vi "QR Code_Example.vi"() -> ()   [LabVIEW 2016]
uses:
  Data Def/QR Code_QR Code Setting.ctl
  <vilib>/vision/Instrument.llb/QR Code Search Options.ctl
  <vilib>/vision/Instrument.llb/Demodulation Mode.ctl
  <vilib>/vision/Instrument.llb/Cell Sample Size.ctl
  <vilib>/vision/Instrument.llb/Cell Filter Mode.ctl
  <vilib>/vision/Instrument.llb/QR Code Description Options.ctl
  <vilib>/vision/Instrument.llb/Data Matrix Polarity.ctl
  <vilib>/vision/Instrument.llb/QR Code Model Type.ctl
  <vilib>/vision/Instrument.llb/QR Code Report.ctl
  <vilib>/vision/Instrument.llb/QR Code Stream Mode Type.ctl
panel:
  out "Time":u32
  out "Data":string
  out "QR Code Report":T1={"Found?"=FALSE, "Data"="", "Bounding Box"=[], "Errors Corrected"=0, "Dimensions (Rows/Cols)"=0, "Version"=0, "QR Model"=0, "Stream Mode"=0, "Barcode Polarity"=-2, "Mirrored?"=FALSE, "Append Stream Position"=0, "Size of Append Stream"=0, "First EAN-128 ID"=0, "First Alternate Language ID"=0, "Append Stream ID"=0, "Minimum Edge Strength"=30, "Demodulation Mode"=-2, "Cell Sample Size"=-2, "Cell Filter Mode"=-2} {"Append Stream ID" format="%x"; "Cell Filter Mode" items=["Auto-detect"=-2, "Average"=0, "Median"=1, "Central Average"=2, "High Average"=3, "Low Average"=4, "Very High Average"=5, "Very Low Average"=6, "All Filters"=8]; "Cell Sample Size" items=["Auto-detect"=-2, "1x1"=1, "2x2"=2, "3x3"=3, "4x4"=4, "5x5"=5, "6x6"=6, "7x7"=7]; "Demodulation Mode" items=["Auto-detect"=-2, "Histogram"=0, "Local Contrast"=1, "Combination"=2, "All"=3]; "Barcode Polarity" items=["Auto-detect"=-2, "Black on White"=0, "White on Black"=1]; "Stream Mode" items=["Numeric", "AlphaNumeric", "Raw Bytes", "UCC/EAN-128 - In Tokens", "UCC/EAN-128 - In Data", "Extended Character Interpretation", "Kanji"]; "QR Model" items=["Auto-detect", "Micro", "Model 1", "Model 2"]; "Version" max=40 step=1}
  in  "Detection":bool
  in  "QR Code Setting":T8={"QR Search Options"={"Rotation Mode"=enum."Unlimited", "Skip Location?"=FALSE, "Edge Threshold"=30, "Demodulation Mode"=-2, "Cell Sample Size"=-2, "Cell Filter Mode"=-2, "Skew Degrees Allowed"=5}, "QR Description Options"={"Matrix Size (cells)"=0, "Barcode Polarity"=-2, "Mirror Mode"=-2, "QR Model"=0}, "QR Code Cell Size (pixels)"={"Minimum Size"=3, "Maximum Size"=7}} {"QR Description Options"."Mirror Mode" items=["Auto-detect"=-2, "Normal"=0, "Mirrored"=1]; "QR Description Options"."Matrix Size (cells)" items=["Auto-detect"=0, "11x11 - Version 1 (Micro QR Only)"=11, "13x13 - Version 2 (Micro QR Only)"=13, "15x15 - Version 3 (Micro QR Only)"=15, "17x17 - Version 4 (Micro QR Only)"=17, "21x21 - Version 1"=21, "25x25 - Version 2"=25, "29x29 - Version 3"=29, "33x33 - Version 4"=33, "37x37 - Version 5"=37, "41x41 - Version 6"=41, "45x45 - Version 7"=45, "49x49 - Version 8"=49, "53x53 - Version 9"=53, "57x57 - Version 10"=57, "61x61 - Version 11"=61, "65x65 - Version 12"=65, "69x69 - Version 13"=69, "73x73 - Version 14"=73, "77x77 - Version 15"=77, "81x81 - Version 16"=81, "85x85 - Version 17"=85, "89x89 - Version 18"=89, "93x93 - Version 19"=93, "97x97 - Version 20"=97, "101x101 - Version 21"=101, "105x105 - Version 22"=105, "109x109 - Version 23"=109, "113x113 - Version 24"=113, "117x117 - Version 25"=117, "121x121 - Version 26"=121, "125x125 - Version 27"=125, "129x129 - Version 28"=129, "133x133 - Version 29"=133, "137x137 - Version 30"=137, "141x141 - Version 31"=141, "145x145 - Version 32"=145, "149x149 - Version 33"=149, "153x153 - Version 34"=153, "157x157 - Version 35"=157, "161x161 - Version 36"=161, "165x165 - Version 37"=165, "169x169 -  Version 38"=169, "173x173 - Version 39"=173, "177x177 - Version 40"=177]; "QR Description Options"."QR Model" items=["Auto-detect", "Micro", "Model 1", "Model 2"]; "QR Description Options"."Barcode Polarity" items=["Auto-detect"=-2, "Black on White"=0, "White on Black"=1]; "QR Search Options"."Cell Filter Mode" items=["Auto-detect"=-2, "Average"=0, "Median"=1, "Central Average"=2, "High Average"=3, "Low Average"=4, "Very High Average"=5, "Very Low Average"=6, "All Filters"=8]; "QR Search Options"."Cell Sample Size" items=["Auto-detect"=-2, "1x1"=1, "2x2"=2, "3x3"=3, "4x4"=4, "5x5"=5, "6x6"=6, "7x7"=7]; "QR Search Options"."Demodulation Mode" items=["Auto-detect"=-2, "Histogram"=0, "Local Contrast"=1, "Combination"=2, "All"=3]}
  out "Image Dst":T11(plugin-control)
  out "Image Src":T11(plugin-control)
  in  "Import Image":bool
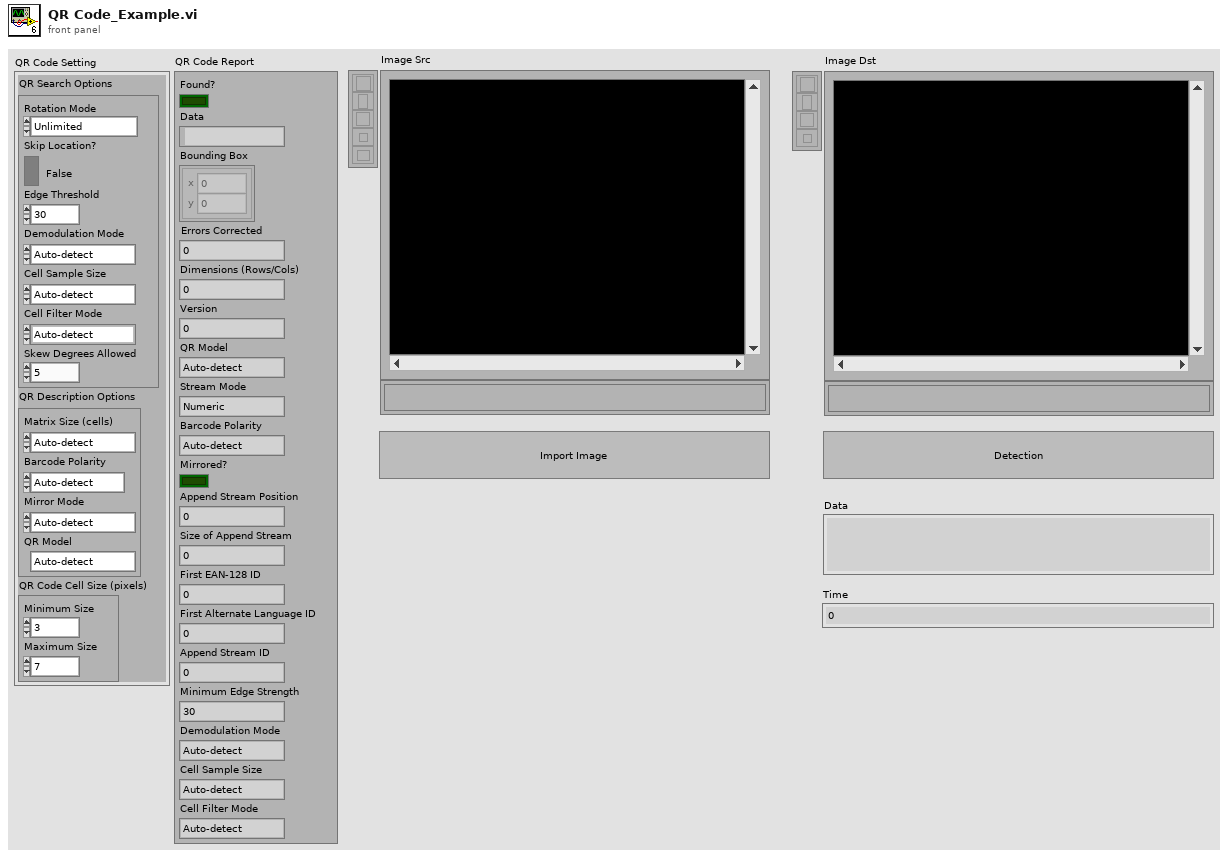
[diagram p1: front panel]
types:
  T1 = typedef "QR Code Report.ctl" = cluster{"Found?":bool, "Data":string, "Bounding Box":cluster{"x":sgl, "y":sgl}[], "Errors Corrected":u32, "Dimensions (Rows/Cols)":u32, "Version":u32, "QR Model":T2, "Stream Mode":T3, "Barcode Polarity":T4, "Mirrored?":bool, "Append Stream Position":u32, "Size of Append Stream":u32, "First EAN-128 ID":i32, "First Alternate Language ID":i32, "Append Stream ID":u32, "Minimum Edge Strength":u32, "Demodulation Mode":T5, "Cell Sample Size":T6, "Cell Filter Mode":T7}
  T2 = typedef "QR Code Model Type.ctl" = i32
  T3 = typedef "QR Code Stream Mode Type.ctl" = i32
  T4 = typedef "Data Matrix Polarity.ctl" = i32
  T5 = typedef "Demodulation Mode.ctl" = i32
  T6 = typedef "Cell Sample Size.ctl" = i32
  T7 = typedef "Cell Filter Mode.ctl" = i32
  T8 = typedef "QR Code_QR Code Setting.ctl" = cluster{"QR Search Options":T9, "QR Description Options":T10, "QR Code Cell Size (pixels)":cluster{"Minimum Size":u32, "Maximum Size":u32}}
  T9 = typedef "QR Code Search Options.ctl" = cluster{"Rotation Mode":enum32{"Unlimited", "0 Degrees", "90 Degrees", "180 Degrees", "270 Degrees"}, "Skip Location?":bool, "Edge Threshold":u32, "Demodulation Mode":T5, "Cell Sample Size":T6, "Cell Filter Mode":T7, "Skew Degrees Allowed":u32}
  T10 = typedef "QR Code Description Options.ctl" = cluster{"Matrix Size (cells)":i32, "Barcode Polarity":T4, "Mirror Mode":i32, "QR Model":T2}
  T11 = typedef "IMAQ Image.ctl" = refnum<image>
  T12 = typedef "QR Code_Buffer Data.ctl" = cluster{"Image Src":T11, "Image Dst":T11, "DVR":refnum<data-value>}
  T13 = cluster{"Global Rectangle":i32[], "Contours":cluster{"Contour Type":u32, "ROI Type":u32, "Points":i32[]}[]}
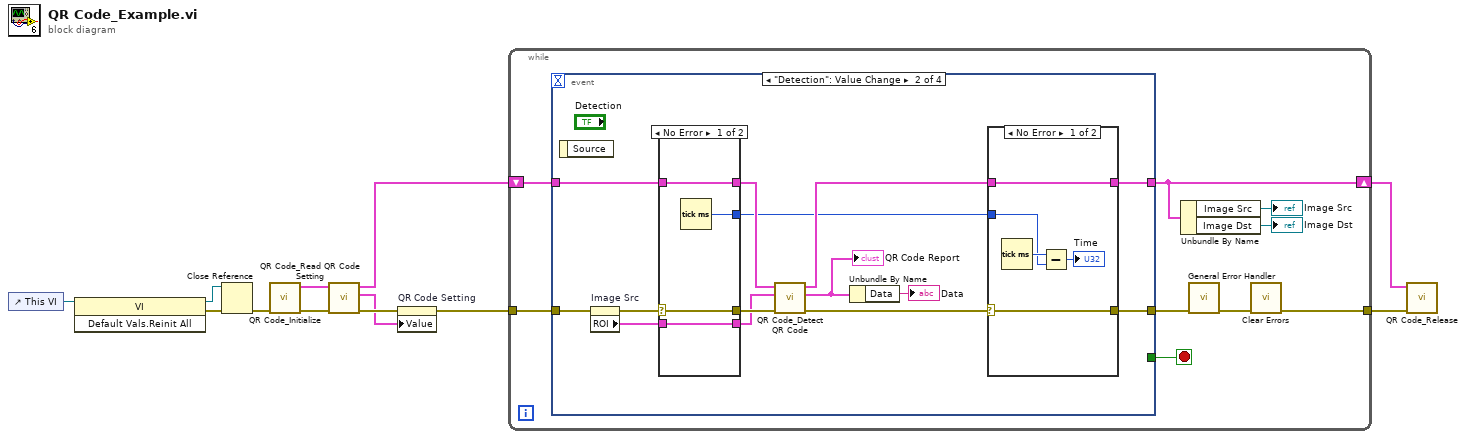
[diagram p0: block diagram]
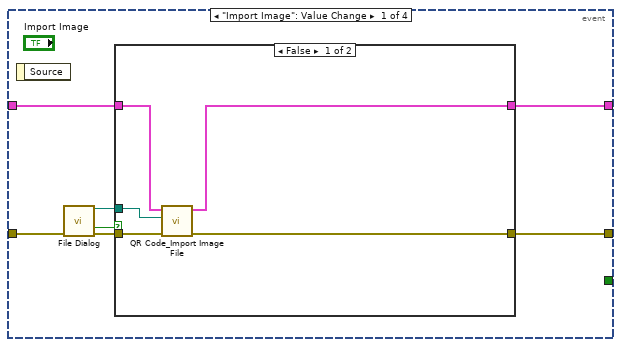
[diagram p2: hidden frame]
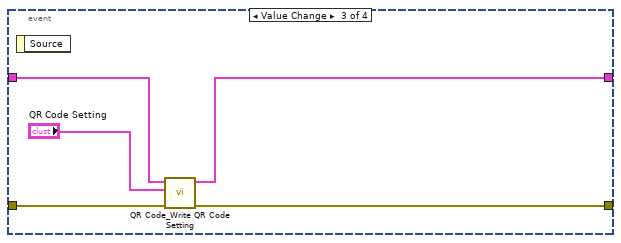
[diagram p6: hidden frame]
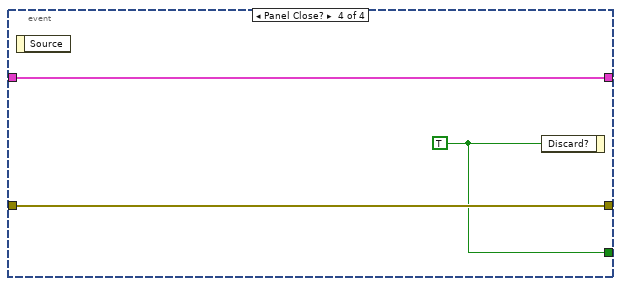
[diagram p7: hidden frame]
diagram:
  n1 = control-ref of="This VI"() -> (w12:refnum<vi>)
  n2 = invoke class="VI" method="Default Vals.Reinit All"(reference=w12) -> (reference out=w10:refnum<vi>, error out=w11:errorcluster)  [unwired: 2 in, 1 out]
  n3 = Close Reference(reference=w10, error in (no error)=w11) -> (error out=w9:errorcluster)
  n4 = call "QR Code_Initialize.vi"("error in"=w9) -> ("error out"=w5:errorcluster, "Buffer Data"=w6:T12)  [unwired: 9 in]
  n5 = call "QR Code_Read QR Code Setting.vi"("error in"=w5, "Buffer Data In"=w6) -> ("error out"=w3:errorcluster, "QR Code Setting"=w2:T8, "Buffer Data Out"=w4:T12)  [unwired: 7 in]
  n6 = property on="QR Code Setting" class="Clust (strict)"(error in=w3, "Value"=w2) -> (error out=w1:errorcluster)  [unwired: 1 in, 1 out]
  n7 = while {
    tunnel: w1 -> [w21]
    shift-right: [w19] -> w7
    shift-left: w4 -> [w20]
    tunnel: [w13] -> w8
    stop <- w16 stop-if-true
    n8 = event shown="[1] \"Detection\": Value Change" {
      selector: _ -> [_ _ _ _]
      dyn-events: _ -> [_ _ _ _]
      timeout: _ -> [_ _ _ _]
      tunnel: w21 -> [w28 w48 w66 w69]
      tunnel: w20 -> [w24 w45 w67 w70]
      tunnel: [w23 w36 w64 w70] -> w19
      tunnel: [w22 w38 w63 w69] -> w15
      tunnel: [_ _ _ w68] -> w16
      event "Import Image": Value Change {
        n9 = event-data() -> ()  [unwired: 1 in, 1 out]
        n10 = call "File Dialog"("error in"=w28) -> ("selected path"=w26:path, "cancelled"=w27:bool, "error out"=w25:errorcluster)  [unwired: 11 in, 1 out]
        n11 = case shown="False" w27 {
          tunnel: w26 -> [w32 _]
          tunnel: w25 -> [w31 _]
          tunnel: w24 -> [w33 w34]
          tunnel: [w30 w34] -> w23
          tunnel: [w29 _] -> w22
          frame False {
            n12 = call "QR Code_Import Image File.vi"("error in"=w31, "File Path"=w32, "Buffer Data In"=w33) -> ("error out"=w29:errorcluster, "Buffer Data Out"=w30:T12)  [unwired: 7 in]
          }
          frame True {
          }
        }
      }
      event "Detection": Value Change {
        n13 = event-data() -> ()  [unwired: 1 in, 1 out]
        n14 = property on="Image Src" class="ImageControl"(error in=w48) -> (error out=w44:errorcluster, "ROI"=w41:T13)  [unwired: 1 in, 1 out]
        n15 = case shown="No Error" w44 {
          selector: w44 -> [w59 w62]
          tunnel: w45 -> [w58 w61]
          tunnel: [w59 w62] -> w43
          tunnel: [w58 w61] -> w42
          tunnel: w41 -> [w57 w60]
          tunnel: [w57 w60] -> w40
          tunnel: [w56 _] -> w35
          frame No Error {
            n16 = Tick Count (ms)() -> (millisecond timer value=w56:u32)
          }
          frame Error {
          }
        }
        n17 = call "QR Code_Detect QR Code.vi"("error in"=w43, "ROI Descriptor"=w40, "Buffer Data In"=w42) -> ("error out"=w39:errorcluster, "QR Code Report"=w47:T1, "Buffer Data Out"=w37:T12)  [unwired: 6 in]
        "QR Code Report" <- w47
        n18 = Unbundle By Name(w47) -> ("Data"=→"Data":string)
        n19 = case shown="No Error" w39 {
          selector: w39 -> [w53 w55]
          tunnel: w37 -> [w52 w54]
          tunnel: [w53 w55] -> w38
          tunnel: [w52 w54] -> w36
          tunnel: w35 -> [w50 _]
          frame No Error {
            n20 = Tick Count (ms)() -> (millisecond timer value=w51:u32)
            n21 = Subtract(x=w51, y=w50) -> (x-y=→"Time":u32)
          }
          frame Error {
          }
        }
      }
      event Value Change {
        n22 = event-data() -> ()  [unwired: 1 in, 1 out]
        n23 = call "QR Code_Write QR Code Setting.vi"("error in"=w66, "QR Code Setting"="QR Code Setting", "Buffer Data In"=w67) -> ("error out"=w63:errorcluster, "Buffer Data Out"=w64:T12)  [unwired: 7 in]
      }
      event Panel Close? {
        w68 = TRUE ("Discard?")
        n24 = event-data() -> ()  [unwired: 1 in, 1 out]
        n25 = event-data("Discard?"=w68) -> ()  [unwired: 1 in, 1 out]
      }
    }
    n26 = Unbundle By Name(w19) -> ("Image Src"=→"Image Src":T11, "Image Dst"=→"Image Dst":T11)
    n27 = call <vilib>:"General Error Handler.vi"("error in (no error)"=w15) -> ("error out"=w14:errorcluster)  [unwired: 10 in, 4 out]
    n28 = call <vilib>:"Clear Errors.vi"("error in (no error)"=w14) -> ("error out"=w13:errorcluster)  [unwired: 5 in, 1 out]
  }
  n29 = call "QR Code_Release.vi"("error in"=w8, "Buffer Data"=w7) -> ()  [unwired: 9 in, 1 out]
